vi "set_TestPoint.vi"() -> ()   [LabVIEW 2014]
panel:
  out "Test Point Written":bool
  out "Dup Aardvark Handle":i32
  out "error out":errorcluster
  in  "error in (no error)":errorcluster
  in  "Address (0x50)":u16=80 max=1023 format="%.0x"
  in  "Aardvark Handle":i32 min=0
  in  "Test Val (V)":dbl
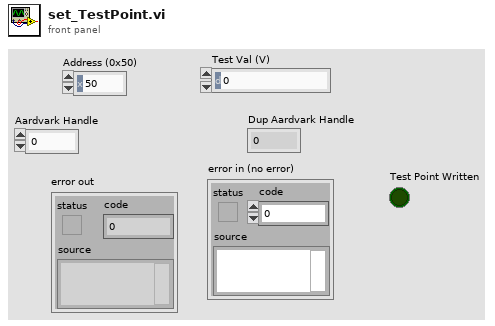
[diagram p1: front panel]
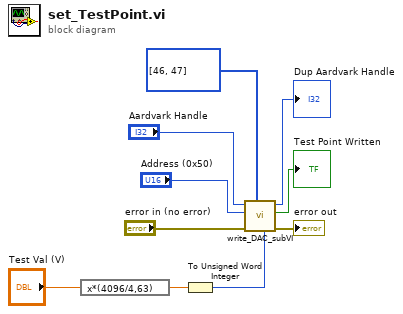
[diagram p0: block diagram]
diagram:
  n1 = expression code="x*(4096/4,63)"("Test Val (V)") -> (w9:dbl)
  n2 = To Unsigned Word Integer(number=w9) -> (unsigned 16bit integer=w8:u16)
  n3 = call "write_DAC_subVI.vi"("Aardvark Handle in"="Aardvark Handle", "Address (0x50) in"="Address (0x50)", "error in (no error)"="error in (no error)", "DAC_ADD"=u8[] [46, 47], "DAC_Val"=w8) -> ("Dup Aardvark Handle"=→"Dup Aardvark Handle":i32, "DAC Written"=→"Test Point Written":bool, "error out"=→"error out":errorcluster)  [unwired: 3 in]
